vi "Util_LoadFileDesriptions.vi"(11 "error in (no error)":errorcluster) -> (1 "Defines":string, 2 "Includes":string, 3 "Compiler Misc Controls":string, 4 "Drop Paths":path[](array[path]), 6 "Drop Files":path[](array[path]), 15 "error out":errorcluster)   [LabVIEW 2011]
doc: "Runs the embedded application on a console located in the <B>Build Path</B> directory ."
uses:
  <vilib>/Utility/config.llb/Read Key (String).vi
  <vilib>/Utility/config.llb/NI_LVConfig.lvlib
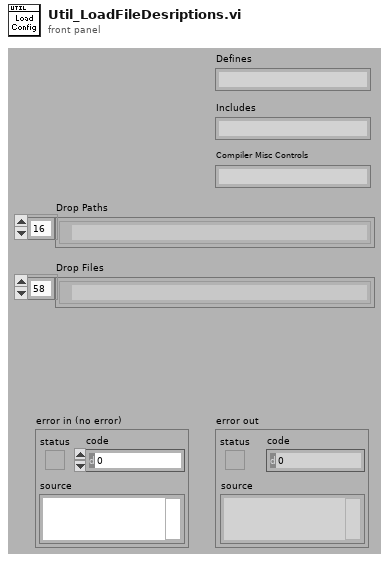
[diagram p1: front panel]
types:
  T1 = typedef "NI_LVConfig.lvlib/Config Data RefNum.ctl" = refnum<k1>
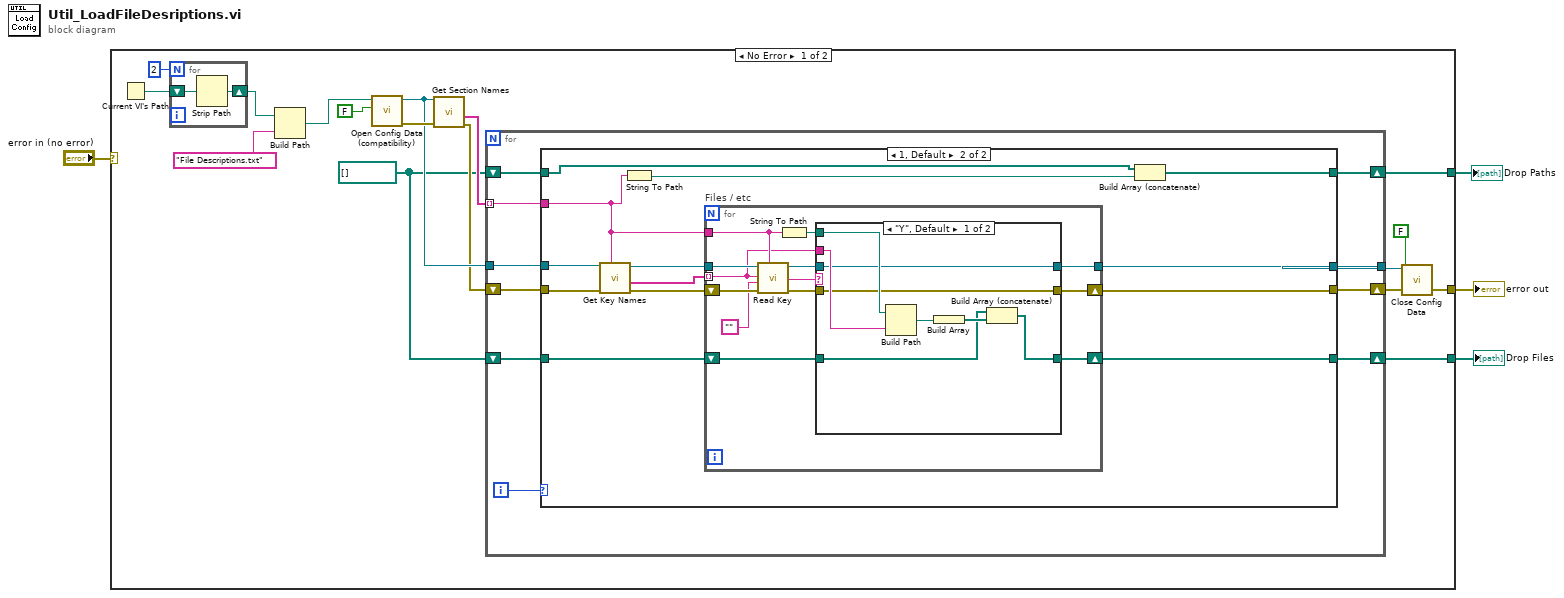
[diagram p0: block diagram]
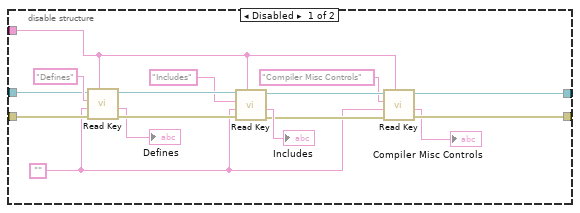
[diagram p3: hidden frame]
diagram:
  n1 = case shown="No Error" "error in (no error)" {
    selector: "error in (no error)" -> [_ w94]
    tunnel: [w14 w94] -> w4
    tunnel: [w17 _] -> w2
    tunnel: [w16 _] -> w1
    frame No Error {
      w12 = path[] []
      n2 = Current VI's Path() -> (path=w10:path)
      n3 = for {
        N: 2 -> [_]
        shift-right: [w22] -> w9
        shift-left: w10 -> [w23]
        n4 = Strip Path(path=w23) -> (stripped path=w22:path)  [unwired: 1 out]
      }
      n5 = Build Path(base path=w9, name or relative path="File Descriptions.txt") -> (appended path=w7:path)
      n6 = call <vilib>:"Open Config Data (compatibility).vi"("create file if necessary (T)"=FALSE ("create file if necessary? (T)"), "configuration file path"=w7) -> ("error out"=w21:errorcluster, "refnum"=w19:T1)  [unwired: 7 in, 1 out]
      n7 = call <vilib>:"Get Section Names.vi"("error in (no error)"=w21, "refnum"=w19) -> ("error out"=w18:errorcluster, "section names"=w20:string[])  [unwired: 7 in, 1 out]
      n8 = for {
        tunnel: w20 -> [w32] mode=indexing
        tunnel: w19 -> [w31]
        shift-right: [w29] -> w15
        shift-left: w18 -> [w30]
        shift-right: [w28] -> w17
        shift-left: w12 -> [w27]
        shift-right: [w26] -> w16
        shift-left: w12 -> [w25]
        tunnel: [w24] -> w13
        i -> [w33]
        n9 = case shown="1, Default" w33 {
          tunnel: w32 -> [w34 w63]
          tunnel: w31 -> [w38 w69]
          tunnel: w30 -> [w37 w68]
          tunnel: [w36 w64] -> w29
          tunnel: [_ w57] -> w28
          tunnel: w27 -> [_ w58]
          tunnel: [_ w61] -> w26
          tunnel: w25 -> [_ w60]
          tunnel: [w35 w59] -> w24
          frame 0 {
            n10 = disable-structure shown="Enabled" {
              disable-tunnel: w38 -> [w50 w56]
              disable-tunnel: w37 -> [w49 w55]
              disable-tunnel: [w44 w55] -> w36
              disable-tunnel: [w41 w56] -> w35
              disable-tunnel: w34 -> [w39 _]
              frame Disabled {
                w43 = ""
                n11 = call-poly <vilib>:"Read Key.vi"("section"=w39, "error in (no error)"=w49, "default value"=w43, "key"="Defines", "refnum"=w50) -> ("error out"=w52:errorcluster, "value"=→"Defines":string, "refnum out"=w53:T1)  [unwired: 3 in, 1 out]
                n12 = call-poly <vilib>:"Read Key.vi"("section"=w39, "error in (no error)"=w52, "default value"=w43, "key"="Includes", "refnum"=w53) -> ("error out"=w45:errorcluster, "value"=→"Includes":string, "refnum out"=w46:T1)  [unwired: 3 in, 1 out]
                n13 = call-poly <vilib>:"Read Key.vi"("section"=w39, "error in (no error)"=w45, "default value"=w43, "key"="Compiler Misc Controls" ("section"), "refnum"=w46) -> ("error out"=w44:errorcluster, "value"=→"Compiler Misc Controls":string, "refnum out"=w41:T1)  [unwired: 3 in, 1 out]
              }
              frame Enabled {
              }
            }
          }
          frame 1, Default {
            n14 = call <vilib>:"Get Key Names.vi"("section"=w63, "error in (no error)"=w68, "refnum"=w69) -> ("error out"=w65:errorcluster, "key names"=w67:string[], "refnum out"=w66:T1)  [unwired: 5 in, 1 out]
            n15 = String To Path(string=w63) -> (path=w62:path)
            n16 = for "Files / etc" {
              tunnel: w63 -> [w80]
              tunnel: w67 -> [w77] mode=indexing
              tunnel: w66 -> [w82]
              shift-right: [w74] -> w64
              shift-left: w65 -> [w81]
              tunnel: [w73] -> w59
              shift-right: [w71] -> w57
              shift-left: w58 -> [w70]
              n17 = call-poly <vilib>:"Read Key.vi"("section"=w80, "error in (no error)"=w81, "default value"="", "key"=w77, "refnum"=w82) -> ("error out"=w75:errorcluster, "value"=w79:string, "refnum out"=w72:T1)  [unwired: 3 in, 1 out]
              n18 = String To Path(string=w80) -> (path=w76:path)
              n19 = case shown="\"Y\", Default" w79 {
                tunnel: w77 -> [w89 _]
                tunnel: w76 -> [w90 _]
                tunnel: w75 -> [w88 w92]
                tunnel: [w88 w92] -> w74
                tunnel: [w87 w91] -> w73
                tunnel: w72 -> [w87 w91]
                tunnel: [w84 w93] -> w71
                tunnel: w70 -> [w83 w93]
                frame "Y", Default {
                  n20 = Build Path(base path=w90, name or relative path=w89) -> (appended path=w86:path)
                  n21 = Build Array(w86) -> (w85:path[])
                  n22 = Build Array (concatenate)(w83, w85) -> (w84:path[])
                }
                frame "N" {
                }
              }
            }
            n23 = Build Array (concatenate)(w60, w62) -> (w61:path[])
          }
        }
      }
      n24 = call <vilib>:"Close Config Data.vi"("error in (no error)"=w15, "write file if changed (T)"=FALSE ("write configuration file? (T)"), "refnum"=w13) -> ("error out"=w14:errorcluster)  [unwired: 7 in, 1 out]
    }
    frame Error {
    }
  }
  "error out" <- w4
  "Drop Paths" <- w1
  "Drop Files" <- w2
